vi "M2p_AD_Std_Sync.vi"() -> ()   [LabVIEW 2015]
uses:
  spcm_library/spcm_gui_common.llb/element_device.ctl
  spcm_library/spcm_gui_m2p.llb/element_m2p_ai_channel.ctl
  spcm_library/spcm_gui_common.llb/element_mode.ctl
  spcm_library/spcm_gui_m2p.llb/element_m2p_ai_trigger.ctl
  spcm_library/spcm_gui_m2p.llb/element_m2p_clock.ctl
  spcm_library/spcm_gui_m2p.llb/element_m2p_ai_multi_purpose_io.ctl
  spcm_library/spcm_gui_common.llb/element_states_rec_sync.ctl
panel:
  in  "Multi IO Lines Settings":T1[](array[typedef]) {"X3 Mode" items=["Disable", "Asynchronous Out", "Asynchronous In", "Trigger Out", "Trigger In", "Clock Out", "Digital In", "Show Run State", "Show Arm State", "Show Sync Arm State"]; "X2 Mode" items=["Disable", "Asynchronous Out", "Asynchronous In", "Trigger Out", "Trigger In", "Clock Out", "Digital In", "Show Run State", "Show Arm State", "Show Sync Arm State"]; "X3 Trigger Mode" items=["Pos. Edge", "Neg. Edge", "Any Edge", "High Level", "Low Level", "PW Long Pos.", "PW Long Neg.", "PW Short Pos.", "PW Short Neg."]; "X2 Trigger Mode" items=["Pos. Edge", "Neg. Edge", "Any Edge", "High Level", "Low Level", "PW Long Pos.", "PW Long Neg.", "PW Short Pos.", "PW Short Neg."]; "X1 Trigger Mode" items=["Pos. Edge", "Neg. Edge", "Any Edge", "High Level", "Low Level", "PW Long Pos.", "PW Long Neg.", "PW Short Pos.", "PW Short Neg."]; "X1 Mode" items=["Disable", "Asynchronous Out", "Asynchronous In", "Trigger Out", "Trigger In", "Clock Out", "Digital In", "Show Run State", "Show Arm State", "Show Sync Arm State"]; "X0 Mode" items=["Disable", "Asynchronous Out", "Trigger Out", "Clock Out", "Show Run State", "Show Arm State", "Show Sync Arm State"]}
  in  "Clock Settings":T2[](array[typedef])=[{"Clock Mode"=0, "Sampling Rate (kHz)"=10000.0, "Clock Output"=FALSE, "Termination"=FALSE, "Ref. Clock (MHz)"=10.0, "Threshold (mV)"=1500}, {"Clock Mode"=0, "Sampling Rate (kHz)"=10000.0, "Clock Output"=FALSE, "Termination"=FALSE, "Ref. Clock (MHz)"=10.0, "Threshold (mV)"=1500}, {"Clock Mode"=0, "Sampling Rate (kHz)"=10000.0, "Clock Output"=FALSE, "Termination"=FALSE, "Ref. Clock (MHz)"=10.0, "Threshold (mV)"=1500}, {"Clock Mode"=0, "Sampling Rate (kHz)"=10000.0, "Clock Output"=FALSE, "Termination"=FALSE, "Ref. Clock (MHz)"=10.0, "Threshold (mV)"=1500}] {"Threshold (mV)" min=-5000 max=5000; "Clock Mode" items=["Internal Clock Quartz", "External Clock", "External Reference Clock"]; "Ref. Clock (MHz)" min=0.0 max=125000.0; "Sampling Rate (kHz)" min=1.0 max=5000000.0}
  in  "Trigger Settings":T3[](array[typedef])=[{"Trigger Source"=0, "External Trigger"=0, "Level 0 Ext"=1500, "Ext Trig Term"=FALSE, "Channel Trigger"=0, "Level 0 Ch"=0, "Level 1 Ch"=0, "Trigger Delay (Samples)"=0}, {"Trigger Source"=0, "External Trigger"=0, "Level 0 Ext"=1500, "Ext Trig Term"=FALSE, "Channel Trigger"=0, "Level 0 Ch"=0, "Level 1 Ch"=0, "Trigger Delay (Samples)"=0}, {"Trigger Source"=0, "External Trigger"=0, "Level 0 Ext"=1500, "Ext Trig Term"=FALSE, "Channel Trigger"=0, "Level 0 Ch"=0, "Level 1 Ch"=0, "Trigger Delay (Samples)"=0}, {"Trigger Source"=0, "External Trigger"=0, "Level 0 Ext"=1500, "Ext Trig Term"=FALSE, "Channel Trigger"=0, "Level 0 Ch"=0, "Level 1 Ch"=0, "Trigger Delay (Samples)"=0}] {"Channel Trigger" items=["None", "Pos. Edge", "Neg. Edge", "Any Edge", "Pos. Rearm", "Neg. Rearm", "Enter Window", "Leave Window", "In Win", "Out Win"]; "External Trigger" items=["None", "Pos. Edge", "Neg. Edge", "Any Edge", "High Level", "Low Level"]; "Trigger Source" items=["Software Trigger", "External Trigger", "Channel 0 Trigger", "Channel 1 Trigger", "Channel 2 Trigger", "Channel 3 Trigger", "Channel 4 Trigger", "Channel 5 Trigger", "Channel 6 Trigger", "Channel 7 Trigger"]; "Trigger Delay (Samples)" max=65535 step=1}
  in  "Mode Settings":T4[](array[typedef])=[{"Mode"=0, "Mem"=16384, "Seg"=1024, "Post"=8192, "Pre"=32, "ABA"=16}, {"Mode"=0, "Mem"=16384, "Seg"=1024, "Post"=8192, "Pre"=32, "ABA"=16}, {"Mode"=0, "Mem"=16384, "Seg"=1024, "Post"=8192, "Pre"=32, "ABA"=16}, {"Mode"=0, "Mem"=16384, "Seg"=1024, "Post"=8192, "Pre"=32, "ABA"=16}] {"Mode" items=["Singleshot", "Multiple Recording", "Gated Sampling", "ABA Mode"]; "ABA" min=2 max=65535 step=1; "Post" min=4 step=4; "Mem" min=8 step=4; "Pre" min=4 max=8176 step=4; "Seg" min=8 step=4}
  in  "Channels Settings":T6(array[cluster])=[{"AI Channel 0"={"Enable"=TRUE, "Input Range "=2, "Termination"=0, "Input Type"=0, "Offset"=0}, "AI Channel 1"={"Enable"=TRUE, "Input Range "=2, "Termination"=0, "Input Type"=0, "Offset"=0}, "AI Channel 2"={"Enable"=TRUE, "Input Range "=2, "Termination"=0, "Input Type"=0, "Offset"=0}, "AI Channel 3"={"Enable"=TRUE, "Input Range "=2, "Termination"=0, "Input Type"=0, "Offset"=0}, "AI Channel 4"={"Enable"=TRUE, "Input Range "=2, "Termination"=0, "Input Type"=0, "Offset"=0}, "AI Channel 5"={"Enable"=TRUE, "Input Range "=2, "Termination"=0, "Input Type"=0, "Offset"=0}, "AI Channel 6"={"Enable"=TRUE, "Input Range "=2, "Termination"=0, "Input Type"=0, "Offset"=0}, "AI Channel 7"={"Enable"=TRUE, "Input Range "=2, "Termination"=0, "Input Type"=0, "Offset"=0}}, {"AI Channel 0"={"Enable"=TRUE, "Input Range "=2, "Termination"=0, "Input Type"=0, "Offset"=0}, "AI Channel 1"={"Enable"=TRUE, "Input Range "=2, "Termination"=0, "Input Type"=0, "Offset"=0}, "AI Channel 2"={"Enable"=TRUE, "Input Range "=2, "Termination"=0, "Input Type"=0, "Offset"=0}, "AI Channel 3"={"Enable"=TRUE, "Input Range "=2, "Termination"=0, "Input Type"=0, "Offset"=0}, "AI Channel 4"={"Enable"=TRUE, "Input Range "=2, "Termination"=0, "Input Type"=0, "Offset"=0}, "AI Channel 5"={"Enable"=TRUE, "Input Range "=2, "Termination"=0, "Input Type"=0, "Offset"=0}, "AI Channel 6"={"Enable"=TRUE, "Input Range "=2, "Termination"=0, "Input Type"=0, "Offset"=0}, "AI Channel 7"={"Enable"=TRUE, "Input Range "=2, "Termination"=0, "Input Type"=0, "Offset"=0}}, {"AI Channel 0"={"Enable"=TRUE, "Input Range "=2, "Termination"=0, "Input Type"=0, "Offset"=0}, "AI Channel 1"={"Enable"=TRUE, "Input Range "=2, "Termination"=0, "Input Type"=0, "Offset"=0}, "AI Channel 2"={"Enable"=TRUE, "Input Range "=2, "Termination"=0, "Input Type"=0, "Offset"=0}, "AI Channel 3"={"Enable"=TRUE, "Input Range "=2, "Termination"=0, "Input Type"=0, "Offset"=0}, "AI Channel 4"={"Enable"=TRUE, "Input Range "=2, "Termination"=0, "Input Type"=0, "Offset"=0}, "AI Channel 5"={"Enable"=TRUE, "Input Range "=2, "Termination"=0, "Input Type"=0, "Offset"=0}, "AI Channel 6"={"Enable"=TRUE, "Input Range "=2, "Termination"=0, "Input Type"=0, "Offset"=0}, "AI Channel 7"={"Enable"=TRUE, "Input Range "=2, "Termination"=0, "Input Type"=0, "Offset"=0}}, {"AI Channel 0"={"Enable"=TRUE, "Input Range "=2, "Termination"=0, "Input Type"=0, "Offset"=0}, "AI Channel 1"={"Enable"=TRUE, "Input Range "=2, "Termination"=0, "Input Type"=0, "Offset"=0}, "AI Channel 2"={"Enable"=TRUE, "Input Range "=2, "Termination"=0, "Input Type"=0, "Offset"=0}, "AI Channel 3"={"Enable"=TRUE, "Input Range "=2, "Termination"=0, "Input Type"=0, "Offset"=0}, "AI Channel 4"={"Enable"=TRUE, "Input Range "=2, "Termination"=0, "Input Type"=0, "Offset"=0}, "AI Channel 5"={"Enable"=TRUE, "Input Range "=2, "Termination"=0, "Input Type"=0, "Offset"=0}, "AI Channel 6"={"Enable"=TRUE, "Input Range "=2, "Termination"=0, "Input Type"=0, "Offset"=0}, "AI Channel 7"={"Enable"=TRUE, "Input Range "=2, "Termination"=0, "Input Type"=0, "Offset"=0}}] {"AI Channel 7"."Input Type" items=["Single-ended", "Differential"]; "AI Channel 7"."Termination" items=["1 MOhm", "50 Ohm"]; "AI Channel 7"."Input Range" items=["±200 mV", "±500 mV", "±1000 mV", "±2000 mV", "±5000 mV", "±10000 mV"]; "AI Channel 6"."Input Type" items=["Single-ended", "Differential"]; "AI Channel 6"."Termination" items=["1 MOhm", "50 Ohm"]; "AI Channel 6"."Input Range" items=["±200 mV", "±500 mV", "±1000 mV", "±2000 mV", "±5000 mV", "±10000 mV"]; "AI Channel 5"."Input Type" items=["Single-ended", "Differential"]; "AI Channel 5"."Termination" items=["1 MOhm", "50 Ohm"]; "AI Channel 5"."Input Range" items=["±200 mV", "±500 mV", "±1000 mV", "±2000 mV", "±5000 mV", "±10000 mV"]; "AI Channel 4"."Input Type" items=["Single-ended", "Differential"]; "AI Channel 4"."Termination" items=["1 MOhm", "50 Ohm"]; "AI Channel 4"."Input Range" items=["±200 mV", "±500 mV", "±1000 mV", "±2000 mV", "±5000 mV", "±10000 mV"]; "AI Channel 3"."Input Type" items=["Single-ended", "Differential"]; "AI Channel 3"."Termination" items=["1 MOhm", "50 Ohm"]; "AI Channel 3"."Input Range" items=["±200 mV", "±500 mV", "±1000 mV", "±2000 mV", "±5000 mV", "±10000 mV"]; "AI Channel 2"."Input Type" items=["Single-ended", "Differential"]; "AI Channel 2"."Termination" items=["1 MOhm", "50 Ohm"]; "AI Channel 2"."Input Range" items=["±200 mV", "±500 mV", "±1000 mV", "±2000 mV", "±5000 mV", "±10000 mV"]; "AI Channel 1"."Input Type" items=["Single-ended", "Differential"]; "AI Channel 1"."Termination" items=["1 MOhm", "50 Ohm"]; "AI Channel 1"."Input Range" items=["±200 mV", "±500 mV", "±1000 mV", "±2000 mV", "±5000 mV", "±10000 mV"]; "AI Channel 0"."Input Type" items=["Single-ended", "Differential"]; "AI Channel 0"."Termination" items=["1 MOhm", "50 Ohm"]; "AI Channel 0"."Input Range" items=["±200 mV", "±500 mV", "±1000 mV", "±2000 mV", "±5000 mV", "±10000 mV"]}
  out "Display Card 3":sgl[][](graph)
  out "Display Card 2":sgl[][](graph)
  out "Display Card 1":sgl[][](graph)
  in  "Select Device to setup":u16(ring) items=["M2p.5962-x4, SN: 100000", "M2p.5962-x4, SN: 100001", "M2p.5962-x4, SN: 100002", "M2p.5962-x4, SN: 100003"]
  out "Status":string="Stopped"
  out "Sync Count":u32=2
  out "Card Infos":T7(array[cluster])=[{"Device Name"="M2p.5968-x4", "Serial Number"=100000.0, "Mem (MB)"=1024.0}, {"Device Name"="M2p.5968-x4", "Serial Number"=100001.0, "Mem (MB)"=1024.0}, {"Device Name"="M2p.5962-x4", "Serial Number"=100002.0, "Mem (MB)"=1024.0}, {"Device Name"="M2p.5962-x4", "Serial Number"=100003.0, "Mem (MB)"=1024.0}]
  in  "Loop Button":bool
  in  "Singleshot Button":bool
  in  "Quit Button":bool
  in  "Stop Button":bool
  out "Display Card 0":sgl[][](graph)
  in  "Device":T8 {"Device" items=["Card", "digitizerNETBOX"]}
  in  "NumCards":u32=2 caption="Number of cards"
  # "Mode"
  # "ASync Write"
  # "Trig-Mode"
  # "Trig-Pulsewidth"
  # "ASync Read"
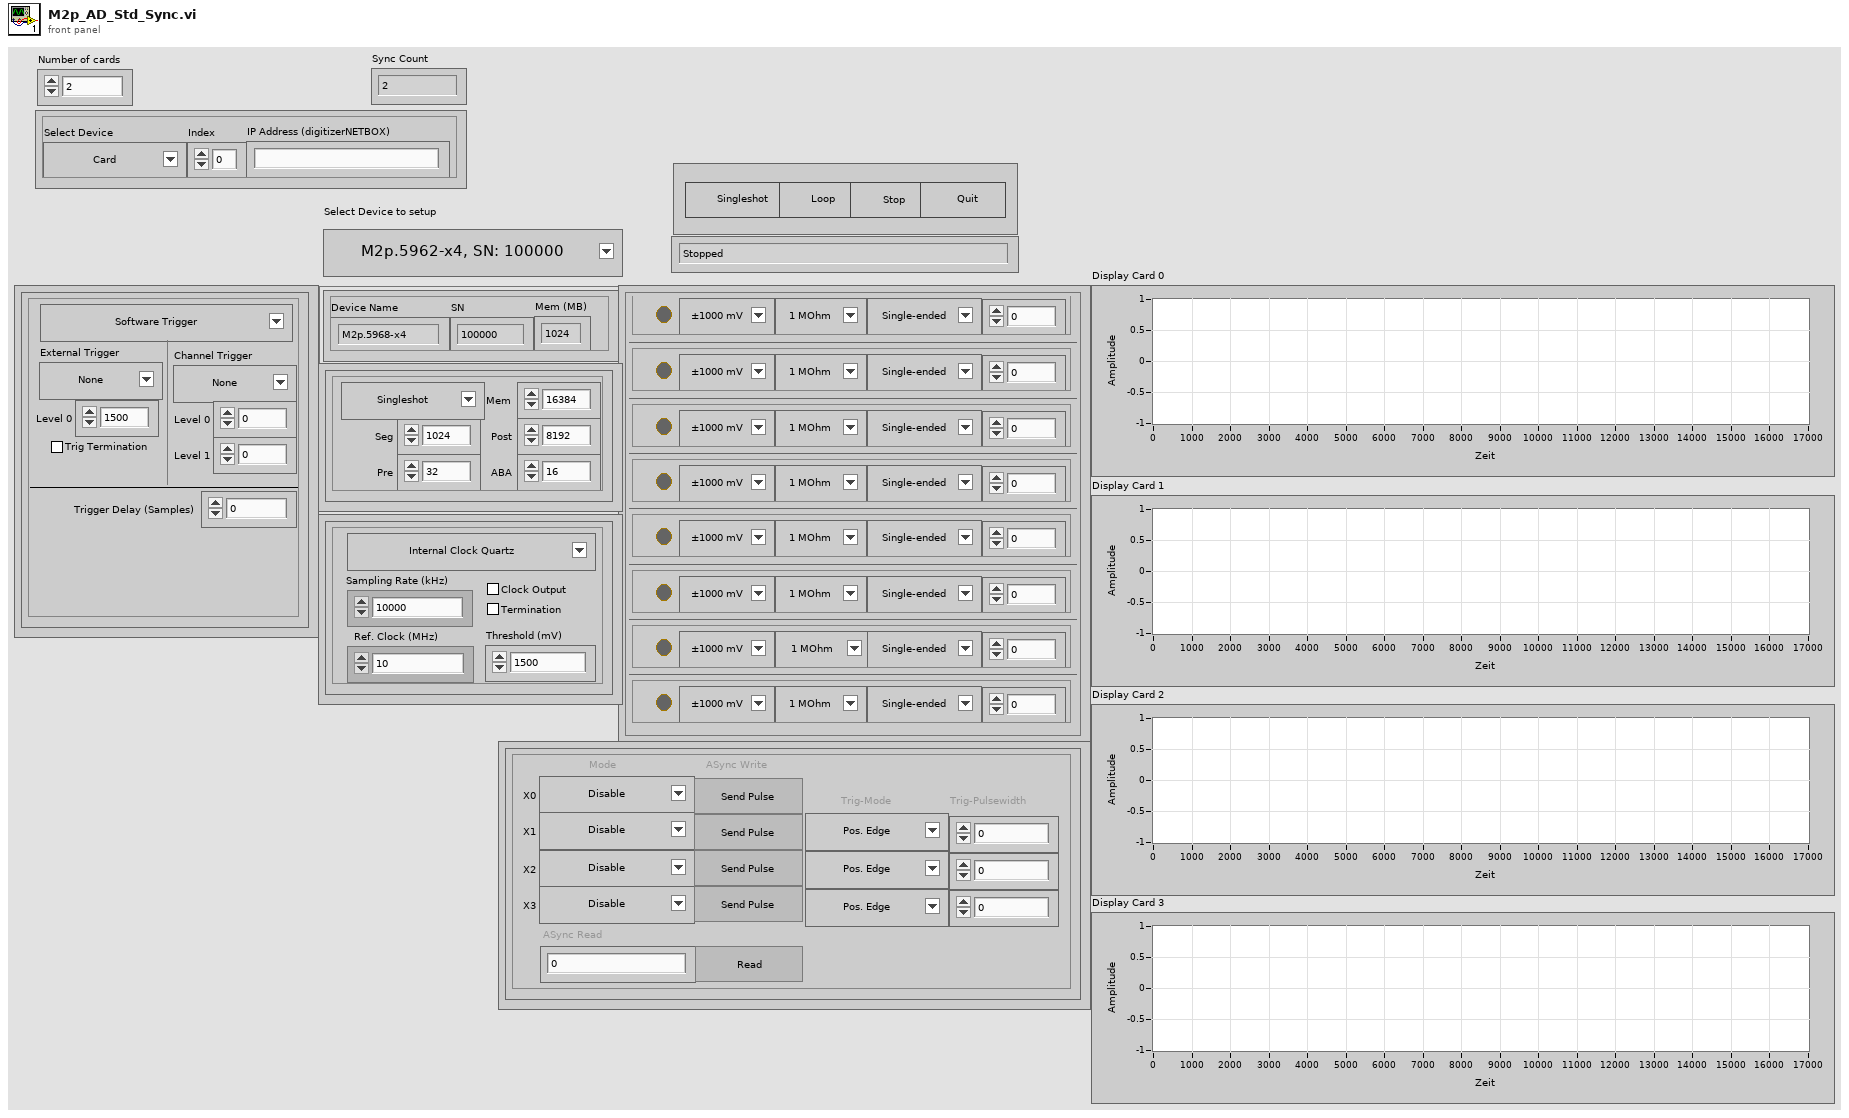
[diagram p1: front panel]
types:
  T1 = typedef "element_m2p_ai_multi_purpose_io.ctl" = cluster{"X0 Mode":u16, "X1 Mode":u16, "X2 Mode":u16, "X3 Mode":u16, "X0 ASync Send Pulse":bool, "X1 ASync Send Pulse":bool, "X2 ASync Send Pulse":bool, "X3 ASync Send Pulse":bool, "X1 Trigger Mode":u16, "X2 Trigger Mode":u16, "X3 Trigger Mode":u16, "X1 Pulsewidth":u32, "X2 Pulsewidth":u32, "X3 Pulsewidth":u32, "ASync Read Button":bool, "ASync Read":i32, "AI":bool}
  T2 = typedef "element_m2p_clock.ctl" = cluster{"Clock Mode":u16, "Sampling Rate (kHz)":dbl, "Clock Output":bool, "Termination":bool, "Ref. Clock (MHz)":dbl, "Threshold (mV)":i32}
  T3 = typedef "element_m2p_ai_trigger.ctl" = cluster{"Trigger Source":u16, "External Trigger":u16, "Level 0 Ext":i32, "Ext Trig Term":bool, "Channel Trigger":u16, "Level 0 Ch":i32, "Level 1 Ch":i32, "Trigger Delay (Samples)":u32}
  T4 = typedef "element_mode.ctl" = cluster{"Mode":u16, "Mem":u32, "Seg":u32, "Post":u32, "Pre":u32, "ABA":u32}
  T5 = typedef "element_m2p_ai_channel.ctl" = cluster{"Enable":bool, "Input Range ":u16, "Termination":u16, "Input Type":u16, "Offset":i32}
  T6 = cluster{"AI Channel 0":T5, "AI Channel 1":T5, "AI Channel 2":T5, "AI Channel 3":T5, "AI Channel 4":T5, "AI Channel 5":T5, "AI Channel 6":T5, "AI Channel 7":T5}[]
  T7 = cluster{"Device Name":string, "Serial Number":dbl, "Mem (MB)":dbl}[]
  T8 = typedef "element_device.ctl" = cluster{"Index":dbl, "IP Address":string, "Device":u16}
  T9 = typedef "element_states_rec_sync.ctl" = enum16{"Idle", "Init GUI", "Init Cards", "Init Sync", "Write Setup", "Start", "Acquire", "Read Data", "Stop", "Close Sync", "Close Cards", "Quit"}
  T10 = enum16{"Idle", "Init", "Write Setup", "Start", "Acquire", "Read Data", "Quit"}
  T11 = cluster{"Device Name":string, "Serial Number":dbl, "Mem (MB)":dbl}
  T12 = cluster{"AI Channel 0":T5, "AI Channel 1":T5, "AI Channel 2":T5, "AI Channel 3":T5, "AI Channel 4":T5, "AI Channel 5":T5, "AI Channel 6":T5, "AI Channel 7":T5}
  T13 = cluster{"Card Type":i32, "Inst Mem (high part)":i32, "Inst Mem (low part)":i32, "Serial Number":i32, "Function Type":i32, "Installed Features":i32, "Base Card Version":i32, "Module Version":i32, "Extension Version":i32, "Production Date":i32, "Max Sampling Rate":i32, "Max Channels":i32, "Demo Card":i32}
  T14 = cluster{"Card Name":string, "SN":i32, "Mem (MB)":i32}
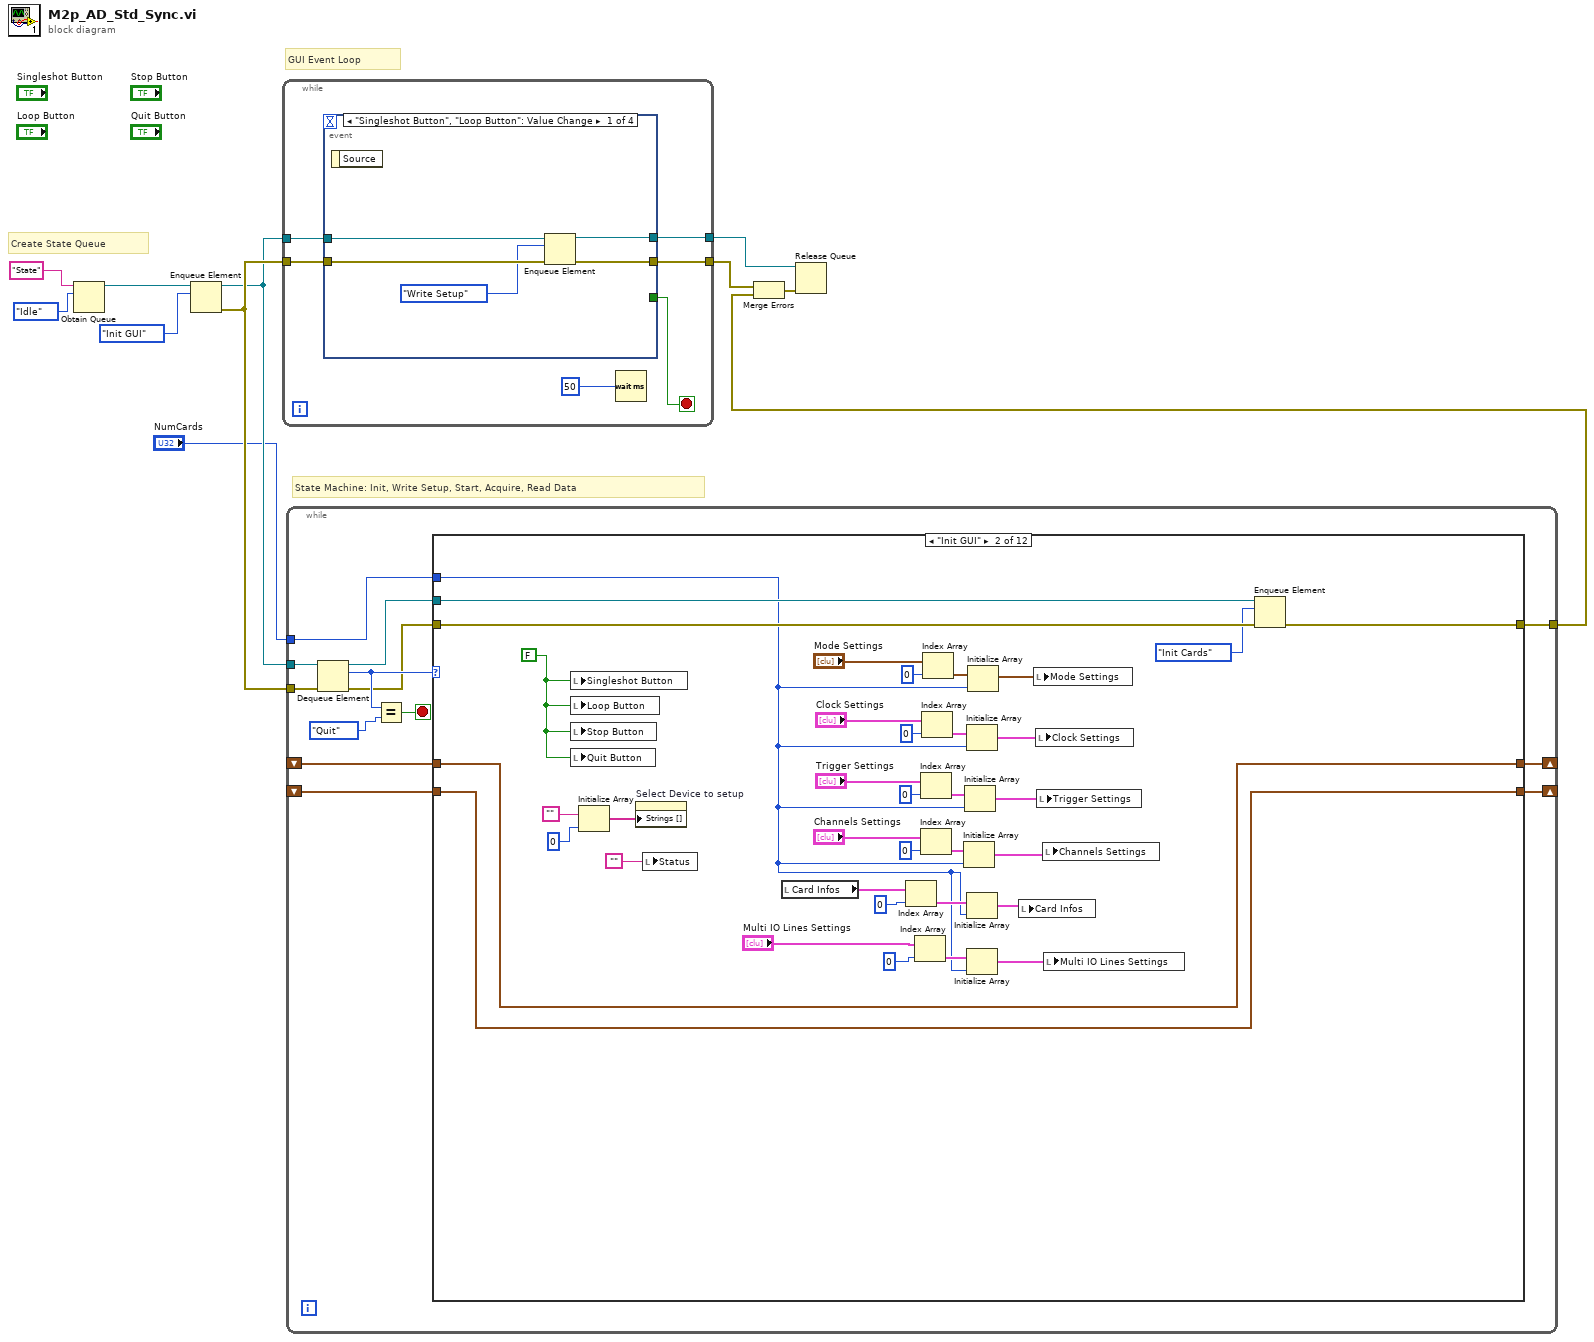
[diagram p0: block diagram]
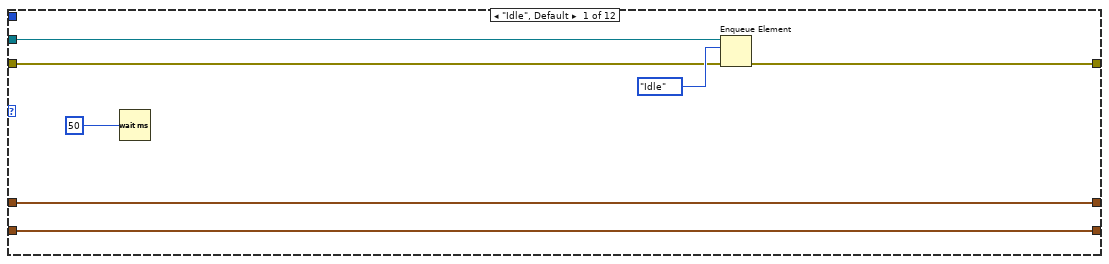
[diagram p2: hidden frame]
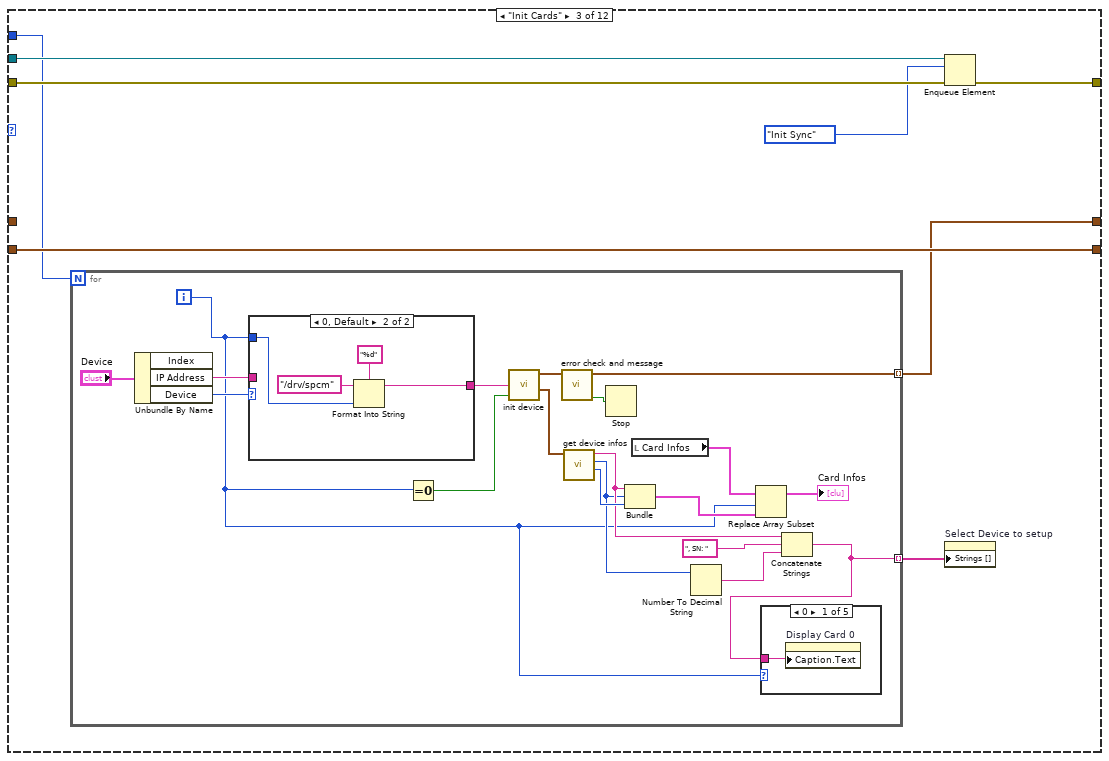
[diagram p3: hidden frame]
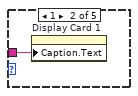
[diagram p4: hidden frame]
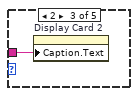
[diagram p5: hidden frame]
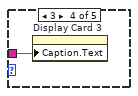
[diagram p6: hidden frame]
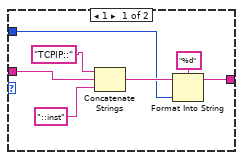
[diagram p8: hidden frame]
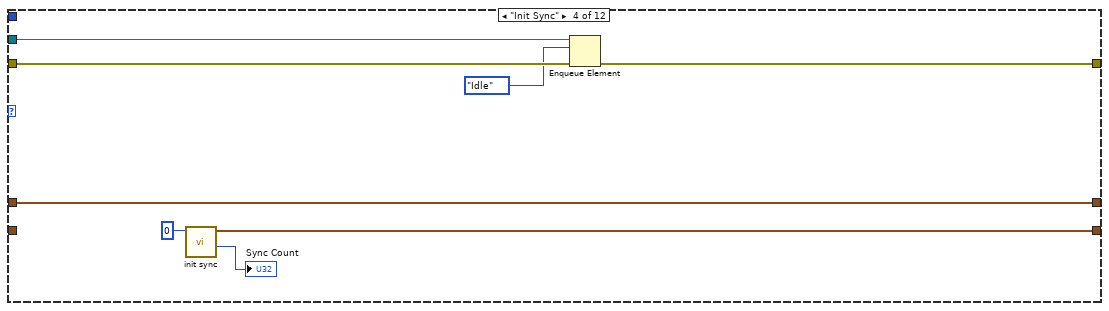
[diagram p9: hidden frame]
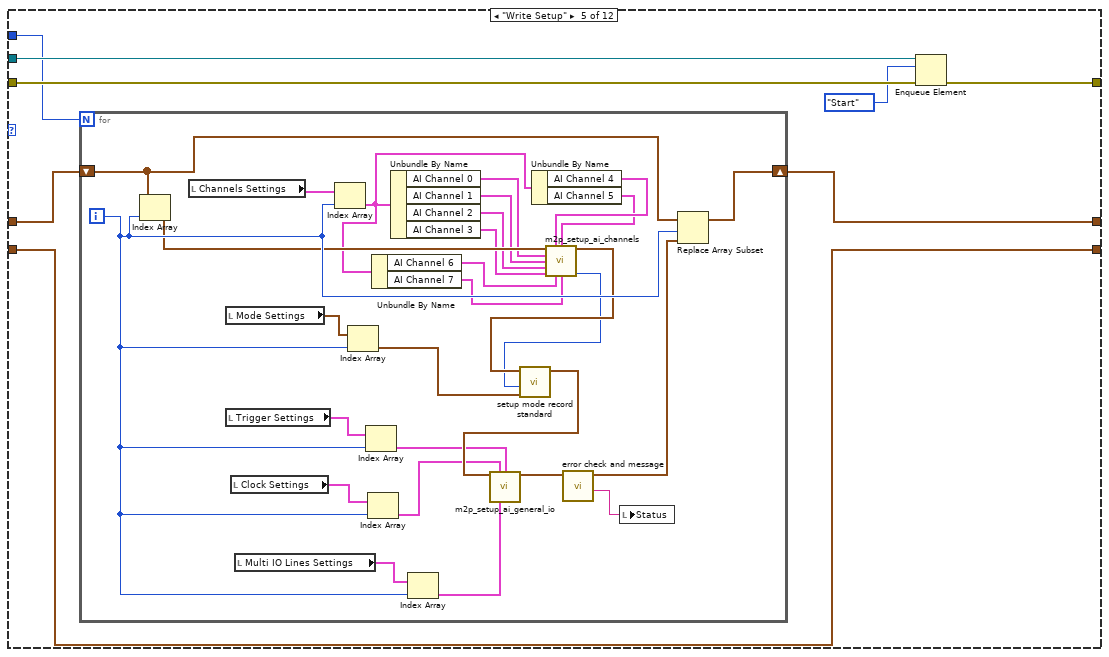
[diagram p10: hidden frame]
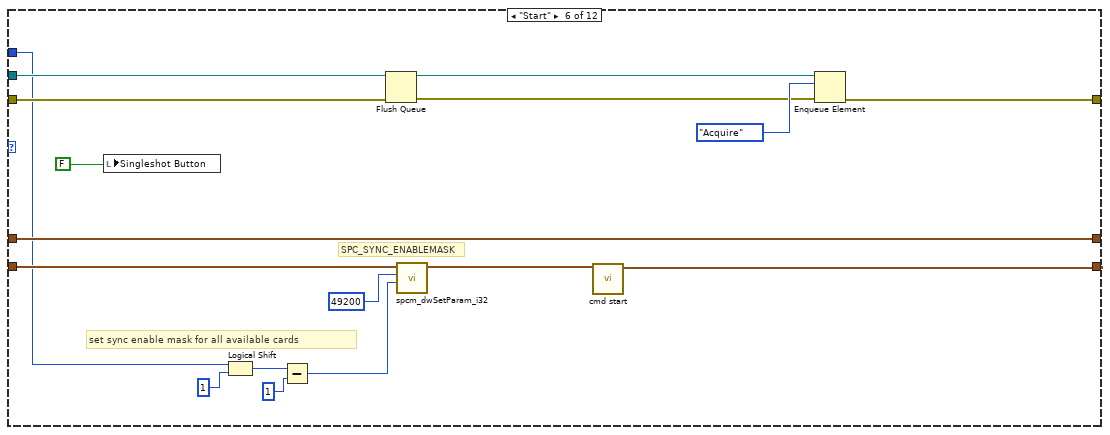
[diagram p11: hidden frame]
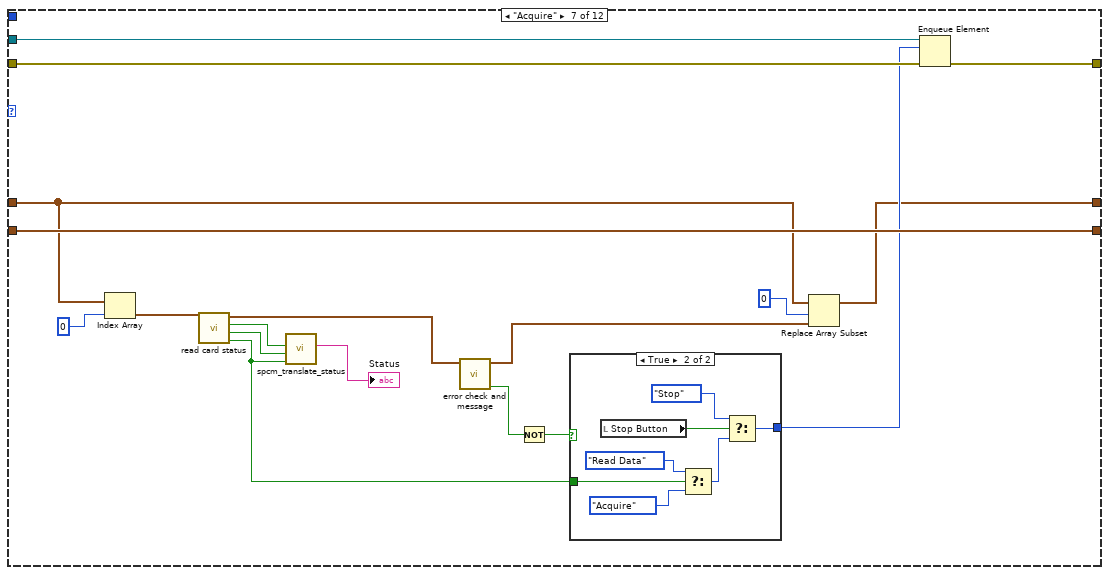
[diagram p12: hidden frame]
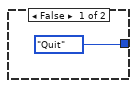
[diagram p13: hidden frame]
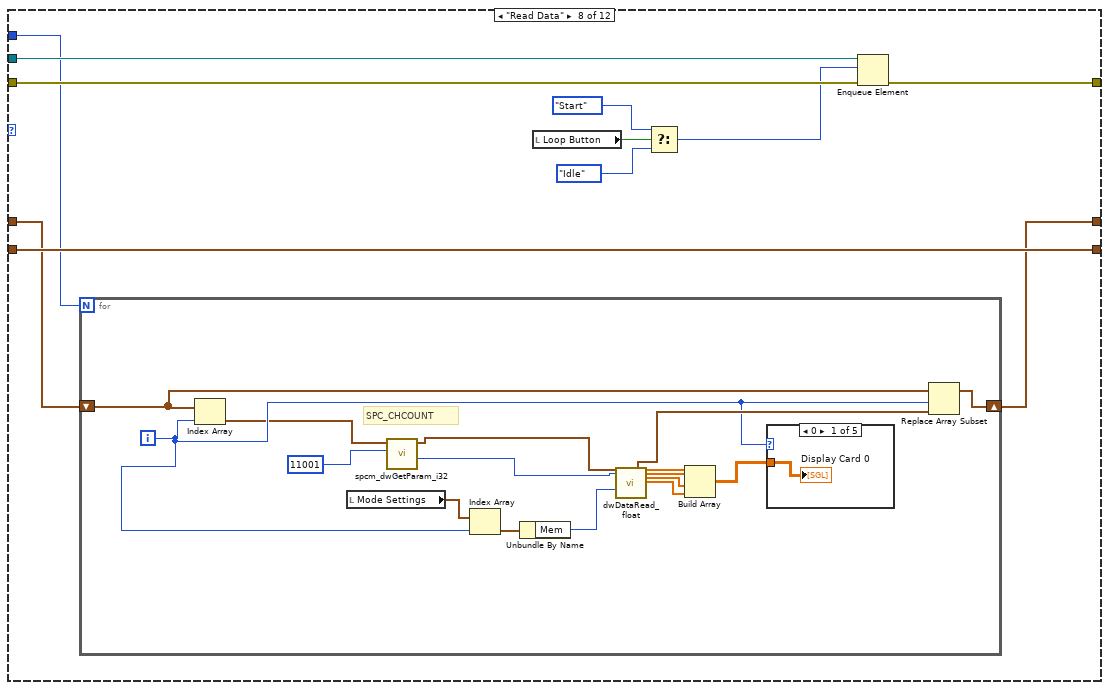
[diagram p14: hidden frame]
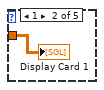
[diagram p15: hidden frame]
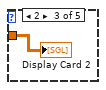
[diagram p16: hidden frame]
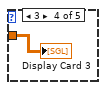
[diagram p17: hidden frame]
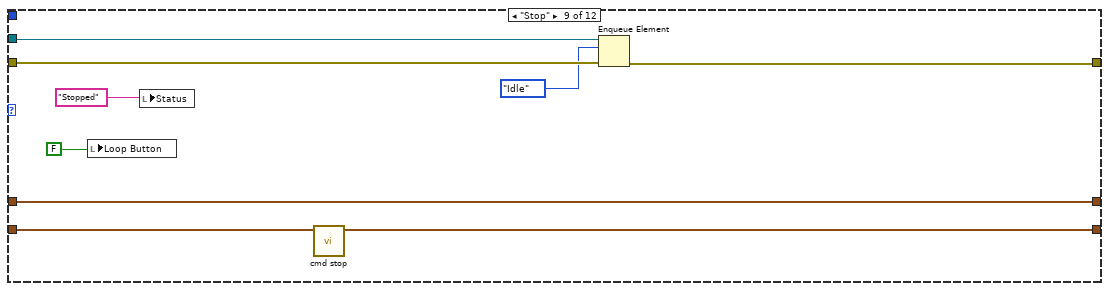
[diagram p19: hidden frame]
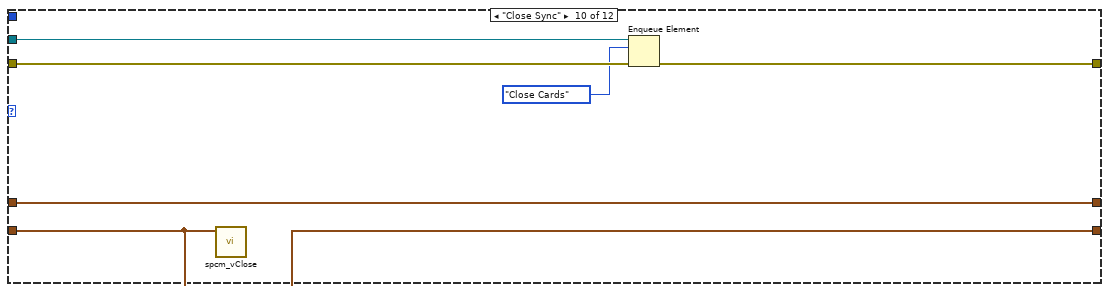
[diagram p20: hidden frame]
diagram:
  # "State Machine: Init, Write Setup, Start, Acquire, Read Data"
  # "GUI Event Loop"
  # "Create State Queue"
  n1 = Obtain Queue(name (unnamed)="State", element data type=element_states_rec_sync."Idle") -> (queue out=w10:refnum<queue>)  [unwired: 3 in, 2 out]
  n2 = Enqueue Element(queue=w10, element=element_states_rec_sync."Init GUI") -> (queue out=w7:refnum<queue>, error out=w8:errorcluster)  [unwired: 2 in, 1 out]
  n3 = while {
    tunnel: w7 -> [w15]
    tunnel: [w16] -> w5
    tunnel: [w12] -> w4
    tunnel: w8 -> [w13]
    stop <- w14 stop-if-true
    n4 = event shown="[0] \"Singleshot Button\", \"Loop Button\": Value Change" {
      selector: _ -> [_ _ _ _]
      dyn-events: _ -> [_ _ _ _]
      timeout: _ -> [_ _ _ _]
      tunnel: [_ _ TRUE _] -> w14
      tunnel: [w22 w27 w32 _] -> w16
      tunnel: w15 -> [w21 w26 w33 _]
      tunnel: [w19 w24 w30 _] -> w12
      tunnel: w13 -> [w20 w25 w29 _]
      event "Singleshot Button", "Loop Button": Value Change {
        n5 = event-data() -> ()  [unwired: 1 in, 1 out]
        n6 = Enqueue Element(queue=w21, element=element_states_rec_sync."Write Setup", error in (no error)=w20) -> (queue out=w22:refnum<queue>, error out=w19:errorcluster)  [unwired: 1 in, 1 out]
      }
      event "Stop Button": Value Change {
        n7 = event-data() -> ()  [unwired: 1 in, 1 out]
        n8 = Enqueue Element(queue=w26, element=element_states_rec_sync."Idle", error in (no error)=w25) -> (queue out=w27:refnum<queue>, error out=w24:errorcluster)  [unwired: 1 in, 1 out]
      }
      event "Quit Button": Value Change {
        n9 = event-data() -> ()  [unwired: 1 in, 1 out]
        n10 = Enqueue Element(queue=w33, element=element_states_rec_sync."Close Sync", error in (no error)=w29) -> (queue out=w32:refnum<queue>, error out=w30:errorcluster)  [unwired: 1 in, 1 out]
      }
      event "Select Device to setup": Value Change {
        n11 = event-data() -> ()  [unwired: 1 in, 1 out]
        n12 = Build Array("Select Device to setup") -> (w34:u16[])
        n13 = property on="Card Infos" class="Arr (strict)"("Index Values"=w34) -> ()  [unwired: 2 in, 2 out]
        n14 = property on="Mode Settings" class="Arr (strict)"("Index Values"=w34) -> ()  [unwired: 2 in, 2 out]
        n15 = property on="Clock Settings" class="Arr (strict)"("Index Values"=w34) -> ()  [unwired: 2 in, 2 out]
        n16 = property on="Trigger Settings" class="Arr (strict)"("Index Values"=w34) -> ()  [unwired: 2 in, 2 out]
        n17 = property on="Multi IO Lines Settings" class="Arr (strict)"("Index Values"=w34) -> ()  [unwired: 2 in, 2 out]
        n18 = property on="Channels Settings" class="Arr (strict)"("Index Values"=w34) -> ()  [unwired: 2 in, 2 out]
      }
    }
    n19 = Wait (ms)(milliseconds to wait=50) -> ()  [unwired: 1 out]
  }
  n20 = while {
    shift-right: [w37] -> _
    shift-left: _ -> [w48]
    tunnel: [w44] -> w3
    tunnel: w8 -> [w43]
    tunnel: w7 -> [w41]
    tunnel: "NumCards" -> [w40]
    shift-right: [w38] -> _
    shift-left: _ -> [w39]
    stop <- w46 stop-if-true
    n21 = Dequeue Element(queue=w41, error in (no error)=w43) -> (queue out=w45:refnum<queue>, element=w47:T9, error out=w42:errorcluster)  [unwired: 1 in, 1 out]
    n22 = Equal?(x=w47, y=element_states_rec_sync."Quit") -> (x = y?=w46:bool)
    n23 = case shown="\"Init GUI\"" w47 {
      tunnel: w48 -> [w55 w68 _ w136 w146 w191 w196 w226 w256 w266 w274 w279]
      tunnel: w45 -> [w50 w91 w99 w141 w149 w184 w212 w231 w260 w265 w272 _]
      tunnel: [w52 w89 w98 w139 w147 w194 w211 w230 w258 w261 w267 w280] -> w44
      tunnel: w42 -> [w49 w90 w96 w140 w148 w186 w210 w229 w259 w264 w271 w280]
      tunnel: w40 -> [_ w69 w94 _ w144 w181 _ w227 _ _ w270 _]
      tunnel: w39 -> [w54 w67 w97 _ w143 w189 w209 w228 w255 w262 w268 w278]
      tunnel: [w54 w67 w97 w135 w143 w193 w209 w228 w254 w262 w268 w278] -> w38
      tunnel: [w55 w68 w92 w136 w145 w191 w195 w223 w256 w266 w273 w279] -> w37
      frame "Idle", Default {
        n24 = Wait (ms)(milliseconds to wait=50) -> ()  [unwired: 1 out]
        n25 = Enqueue Element(queue=w50, element=element_states_rec_sync."Idle", error in (no error)=w49) -> (error out=w52:errorcluster)  [unwired: 1 in, 2 out]
      }
      frame "Init GUI" {
        w88 = FALSE
        n26 = local write "Singleshot Button"(w88) -> ()
        n27 = local write "Loop Button"(w88) -> ()
        n28 = local write "Stop Button"(w88) -> ()
        n29 = local write "Quit Button"(w88) -> ()
        n30 = Initialize Array("", 0) -> (w85:string[])
        n31 = property on="Select Device to setup" class="Ring (strict)"("Strings []"=w85) -> ()  [unwired: 2 in, 2 out]
        n32 = local write "Status"("") -> ()
        n33 = local read "Card Infos"() -> (w83:T7)
        n34 = Index Array(array=w83, index=0) -> (element=w82:T11)
        n35 = Index Array(array="Multi IO Lines Settings", index=0) -> (element=w71:T1)
        n36 = Index Array(array="Trigger Settings", index=0) -> (element=w78:T3)
        n37 = Index Array(array="Channels Settings", index=0) -> (element=w79:T12)
        n38 = Index Array(array="Clock Settings", index=0) -> (element=w75:T2)
        n39 = Index Array(array="Mode Settings", index=0) -> (element=w74:T4)
        n40 = Initialize Array(w79, w69) -> (w58:T6)
        n41 = Initialize Array(w78, w69) -> (w59:T3[])
        n42 = Initialize Array(w75, w69) -> (w60:T2[])
        n43 = Initialize Array(w82, w69) -> (w81:T7)
        n44 = Initialize Array(w71, w69) -> (w56:T1[])
        n45 = Initialize Array(w74, w69) -> (w61:T4[])
        n46 = local write "Card Infos"(w81) -> ()
        n47 = local write "Mode Settings"(w61) -> ()
        n48 = local write "Clock Settings"(w60) -> ()
        n49 = local write "Trigger Settings"(w59) -> ()
        n50 = local write "Channels Settings"(w58) -> ()
        n51 = local write "Multi IO Lines Settings"(w56) -> ()
        n52 = Enqueue Element(queue=w91, element=element_states_rec_sync."Init Cards", error in (no error)=w90) -> (error out=w89:errorcluster)  [unwired: 1 in, 2 out]
      }
      frame "Init Cards" {
        n53 = for {
          N: w94 -> [_]
          tunnel: [w100] -> w92 mode=indexing
          tunnel: [w103] -> w93 mode=indexing
          i -> [w102]
          n54 = Unbundle By Name("Device") -> ("IP Address"=w117:string, "Device"=w116:u16)  [unwired: 1 out]
          n55 = case shown="0, Default" w116 {
            tunnel: w117 -> [w129 _]
            tunnel: [w124 w131] -> w115
            tunnel: w102 -> [w123 w130]
            frame 1 {
              n56 = Concatenate Strings("TCPIP::", w129, "::inst") -> (w125:string)
              n57 = Format Into String(format string="%d", initial string=w125, w123) -> (resulting string=w124:string)  [unwired: 1 in, 1 out]
            }
            frame 0, Default {
              n58 = Format Into String(format string="%d", initial string="/drv/spcm", w130) -> (resulting string=w131:string)  [unwired: 1 in, 1 out]
            }
          }
          n59 = Equal To 0?(x=w102) -> (x = 0?=w101:bool)
          n60 = call "init device.vi"("Device String"=w115, "Free All Devices"=w101) -> ("Card Info Out"=w113:cluster{"Card Handle":u64, "Error Code":u32}, "Card Information"=w112:T13)  [unwired: 3 in]
          n61 = call "error check and message.vi"("Card Info In"=w113) -> ("Error occurred"=w114:bool, "Card Info Out"=w100:cluster{"Card Handle":u64, "Error Code":u32})  [unwired: 4 in, 1 out]
          n62 = call "get device infos.vi"("Card Information"=w112) -> ("Mem (MB)"=w111:i32, "SN"=w106:i32, "Card Name"=w107:string)  [unwired: 8 in]
          n63 = Stop(stop? (T)=w114) -> ()
          n64 = Bundle("Card Name"=w107, "SN"=w106, "Mem (MB)"=w111) -> (w109:T14)  [unwired: 1 in]
          n65 = local read "Card Infos"() -> (w110:T7)
          n66 = Number To Decimal String(number=w106) -> (decimal integer string=w104:string)  [unwired: 1 in]
          n67 = Replace Array Subset(array=w110, new element=w109, index=w102) -> (→"Card Infos":T7)
          n68 = Concatenate Strings(w107, ", SN: ", w104) -> (w103:string)
          n69 = case shown="0" w102 {
            tunnel: w103 -> [w119 w120 w121 w122 _]
            frame 0 {
              n70 = property on="Display Card 0" class="WFGraph (strict)"("Caption.Text"=w119) -> ()  [unwired: 2 in, 2 out]
            }
            frame 1 {
              n71 = property on="Display Card 1" class="WFGraph (strict)"("Caption.Text"=w120) -> ()  [unwired: 2 in, 2 out]
            }
            frame 2 {
              n72 = property on="Display Card 2" class="WFGraph (strict)"("Caption.Text"=w121) -> ()  [unwired: 2 in, 2 out]
            }
            frame 3 {
              n73 = property on="Display Card 3" class="WFGraph (strict)"("Caption.Text"=w122) -> ()  [unwired: 2 in, 2 out]
            }
            frame 4, Default {
            }
          }
        }
        n74 = Enqueue Element(queue=w99, element=element_states_rec_sync."Init Sync", error in (no error)=w96) -> (error out=w98:errorcluster)  [unwired: 1 in, 2 out]
        n75 = property on="Select Device to setup" class="Ring (strict)"("Strings []"=w93) -> ()  [unwired: 2 in, 2 out]
      }
      frame "Init Sync" {
        n76 = call "init sync.vi"("Sync Index"=u32 0 ("Card Index")) -> ("Sync count"=→"Sync Count":i32, "Sync Info Out"=w135:cluster{"Sync Handle":u64, "Error Code":u32})  [unwired: 5 in]
        n77 = Enqueue Element(queue=w141, element=element_states_rec_sync."Idle", error in (no error)=w140) -> (error out=w139:errorcluster)  [unwired: 1 in, 2 out]
      }
      frame "Write Setup" {
        n78 = for {
          N: w144 -> [_]
          shift-right: [w173] -> w145
          shift-left: w146 -> [w174]
          i -> [w175]
          n79 = Index Array(array=w174, index=w175) -> (element=w171:cluster{"Card Handle":u64, "Error Code":u32})
          n80 = local read "Channels Settings"() -> (w168:T6)
          n81 = local read "Mode Settings"() -> (w159:T4[])
          n82 = local read "Trigger Settings"() -> (w156:T3[])
          n83 = local read "Clock Settings"() -> (w155:T2[])
          n84 = local read "Multi IO Lines Settings"() -> (w154:T1[])
          n85 = Index Array(array=w168, index=w175) -> (element=w150:T12)
          n86 = Index Array(array=w159, index=w175) -> (element=w177:T4)
          n87 = Index Array(array=w156, index=w175) -> (element=w153:T3)
          n88 = Index Array(array=w155, index=w175) -> (element=w152:T2)
          n89 = Unbundle By Name(w150) -> ("AI Channel 6"=w161:T5, "AI Channel 7"=w160:T5)
          n90 = Unbundle By Name(w150) -> ("AI Channel 0"=w167:T5, "AI Channel 1"=w166:T5, "AI Channel 2"=w165:T5, "AI Channel 3"=w164:T5)
          n91 = Index Array(array=w154, index=w175) -> (element=w151:T1)
          n92 = Unbundle By Name(w150) -> ("AI Channel 4"=w163:T5, "AI Channel 5"=w162:T5)
          n93 = call "m2p_setup_ai_channels.vi"("Card Info In"=w171, "AI Channel 4"=w163, "AI Channel 5"=w162, "AI Channel 0"=w167, "AI Channel 1"=w166, "AI Channel 2"=w165, "AI Channel 3"=w164, "AI Channel 6"=w161, "AI Channel 7"=w160) -> ("Card Info Out"=w170:cluster{"Card Handle":u64, "Error Code":u32}, "ChMask"=w169:i32)  [unwired: 5 in]
          n94 = call "setup mode record standard.vi"("Mode Setup"=w177, "Channel Mask Low"=w169, "Card Info In"=w170) -> ("Card Info Out"=w157:cluster{"Card Handle":u64, "Error Code":u32})  [unwired: 3 in, 1 out]
          n95 = call "m2p_setup_ai_general_io.vi"("Card Info In"=w157, "Clock Settings"=w152, "Trigger Settings"=w153, "Multi Purpose IO Lines"=w151) -> ("Card Info Out"=w158:cluster{"Card Handle":u64, "Error Code":u32})  [unwired: 8 in, 3 out]
          n96 = call "error check and message.vi"("Card Info In"=w158) -> ("Error Message"=w172:string, "Card Info Out"=w176:cluster{"Card Handle":u64, "Error Code":u32})  [unwired: 4 in, 1 out]
          n97 = local write "Status"(w172) -> ()
          n98 = Replace Array Subset(array=w174, new element=w176, index=w175) -> (w173:cluster{"Card Handle":u64, "Error Code":u32}[])
        }
        n99 = Enqueue Element(queue=w149, element=element_states_rec_sync."Start", error in (no error)=w148) -> (error out=w147:errorcluster)  [unwired: 1 in, 2 out]
      }
      frame "Start" {
        # "set sync enable mask for all available cards"
        # "SPC_SYNC_ENABLEMASK"
        n100 = local write "Singleshot Button"(FALSE) -> ()
        n101 = Logical Shift(y=w181, x=1) -> (x << y=w180:i32)
        n102 = Subtract(x=w180, y=1) -> (x-y=w178:i32)
        n103 = Flush Queue(queue=w184, error in (no error)=w186) -> (queue out=w183:refnum<queue>, error out=w185:errorcluster)  [unwired: 1 out]
        n104 = call "spcm_dwSetParam_i32.vi"("Value (int32)"=w178, "Register"=49200, "Card Info In"=w189) -> ("Card Info Out"=w188:cluster{"Card Handle":u64, "Error Code":u32})  [unwired: 4 in]
        n105 = call "cmd start.vi"("Card Info In"=w188) -> ("Card Info Out"=w193:cluster{"Card Handle":u64, "Error Code":u32})  [unwired: 6 in]
        n106 = Enqueue Element(queue=w183, element=element_states_rec_sync."Acquire", error in (no error)=w185) -> (error out=w194:errorcluster)  [unwired: 1 in, 2 out]
      }
      frame "Acquire" {
        n107 = Index Array(array=w196, index=0) -> (element=w205:cluster{"Card Handle":u64, "Error Code":u32})
        n108 = call "read card status.vi"("Card Info In"=w205) -> ("Card ready"=w200:bool, "Trigger detected"=w207:bool, "Pretrigger full"=w206:bool, "Card Info Out"=w203:cluster{"Card Handle":u64, "Error Code":u32})  [unwired: 3 in]
        n109 = call "spcm_translate_status.vi"("Ready"=w200, "Trigger"=w207, "Pretrigger"=w206) -> ("Text"=→"Status":string)  [unwired: 4 in]
        n110 = call "error check and message.vi"("Card Info In"=w203) -> ("Error occurred"=w202:bool, "Card Info Out"=w198:cluster{"Card Handle":u64, "Error Code":u32})  [unwired: 4 in, 1 out]
        n111 = Not(x=w202) -> (.not. x?=w201:bool)
        n112 = case shown="True" w201 {
          tunnel: [T10."Quit" w220] -> w199
          tunnel: w200 -> [_ w218]
          frame False {
          }
          frame True {
            n113 = local read "Stop Button"() -> (w217:bool)
            n114 = Select(t=element_states_rec_sync."Read Data", s=w218, f=element_states_rec_sync."Acquire") -> (s? t:f=w219:T9)
            n115 = Select(t=element_states_rec_sync."Stop", s=w217, f=w219) -> (s? t:f=w220:T9)
          }
        }
        n116 = Replace Array Subset(array=w196, new element=w198, index=0) -> (w195:cluster{"Card Handle":u64, "Error Code":u32}[])
        n117 = Enqueue Element(queue=w212, element=w199, error in (no error)=w210) -> (error out=w211:errorcluster)  [unwired: 1 in, 2 out]
      }
      frame "Read Data" {
        n118 = for {
          N: w227 -> [_]
          shift-right: [w243] -> w223
          shift-left: w226 -> [w244]
          i -> [w239]
          # "SPC_CHCOUNT"
          n119 = Index Array(array=w244, index=w239) -> (element=w236:cluster{"Card Handle":u64, "Error Code":u32})
          n120 = local read "Mode Settings"() -> (w232:T4[])
          n121 = call "spcm_dwGetParam_i32.vi"("Register"=11001, "Card Info In"=w236) -> ("Value (int32)"=w233:i32, "Card Info Out"=w235:cluster{"Card Handle":u64, "Error Code":u32})  [unwired: 4 in]
          n122 = Index Array(array=w232, index=w239) -> (element=w247:T4)
          n123 = Unbundle By Name(w247) -> ("Mem"=w246:u32)
          n124 = call "dwDataRead_float.vi"("Card Info In"=w235, "Channel Count"=w233, "Length (Samples per Channel)"=w246) -> ("Card Info Out"=w245:cluster{"Card Handle":u64, "Error Code":u32}, "Ch 0"=w242:sgl[], "Ch 1"=w241:sgl[], "Ch 2"=w240:sgl[], "Ch 3"=w238:sgl[])  [unwired: 8 in, 12 out]
          n125 = Build Array(w242, w241, w240, w238) -> (w237:sgl[][])
          n126 = case shown="0" w239 {
            tunnel: w237 -> [w248 w249 w250 w251 _]
            frame 0 {
              "Display Card 0" <- w248
            }
            frame 1 {
              "Display Card 1" <- w249
            }
            frame 2 {
              "Display Card 2" <- w250
            }
            frame 3 {
              "Display Card 3" <- w251
            }
            frame 4, Default {
            }
          }
          n127 = Replace Array Subset(array=w244, new element=w245, index=w239) -> (w243:cluster{"Card Handle":u64, "Error Code":u32}[])
        }
        n128 = local read "Loop Button"() -> (w225:bool)
        n129 = Select(t=element_states_rec_sync."Start", s=w225, f=element_states_rec_sync."Idle") -> (s? t:f=w224:T9)
        n130 = Enqueue Element(queue=w231, element=w224, error in (no error)=w229) -> (error out=w230:errorcluster)  [unwired: 1 in, 2 out]
      }
      frame "Stop" {
        n131 = local write "Loop Button"(FALSE) -> ()
        n132 = local write "Status"("Stopped") -> ()
        n133 = call "cmd stop.vi"("Card Info In"=w255) -> ("Card Info Out"=w254:cluster{"Card Handle":u64, "Error Code":u32})  [unwired: 6 in]
        n134 = Enqueue Element(queue=w260, element=element_states_rec_sync."Idle", error in (no error)=w259) -> (error out=w258:errorcluster)  [unwired: 1 in, 2 out]
      }
      frame "Close Sync" {
        n135 = call "spcm_vClose.vi"("Card Info In"=w262) -> ()  [unwired: 7 in]
        n136 = Enqueue Element(queue=w265, element=element_states_rec_sync."Close Cards", error in (no error)=w264) -> (error out=w261:errorcluster)  [unwired: 1 in, 2 out]
      }
      frame "Close Cards" {
        n137 = for {
          N: w270 -> [_]
          shift-right: [w276] -> w273
          shift-left: w274 -> [w276]
          i -> [w277]
          n138 = Index Array(array=w276, index=w277) -> (element=w275:cluster{"Card Handle":u64, "Error Code":u32})
          n139 = call "spcm_vClose.vi"("Card Info In"=w275) -> ()  [unwired: 7 in]
        }
        n140 = Enqueue Element(queue=w272, element=element_states_rec_sync."Quit", error in (no error)=w271) -> (error out=w267:errorcluster)  [unwired: 1 in, 2 out]
      }
      frame "Quit" {
      }
    }
  }
  n141 = Merge Errors(w4, w3) -> (w6:errorcluster)
  n142 = Release Queue(queue=w5, error in (no error)=w6) -> ()  [unwired: 1 in, 3 out]
